vi "Progetto_AnalisiDimensionale_new.vi"() -> ()   [LabVIEW 2020]
panel:
  out "Write Error":errorcluster
  out "data":string[][](array[string])
  out "Read Error":errorcluster
  in  "Saving File Path":path
  out "Alarm":bool
  out "Length [mm]":dbl
  out "Speed [m/s]":dbl
  in  "Sensors_Distance [mm]":u32=101
  in  "Max_Time [ms]":u32
  in  "Trigger_S2":bool
  in  "Trigger_S1":bool
  in  "STOP":bool
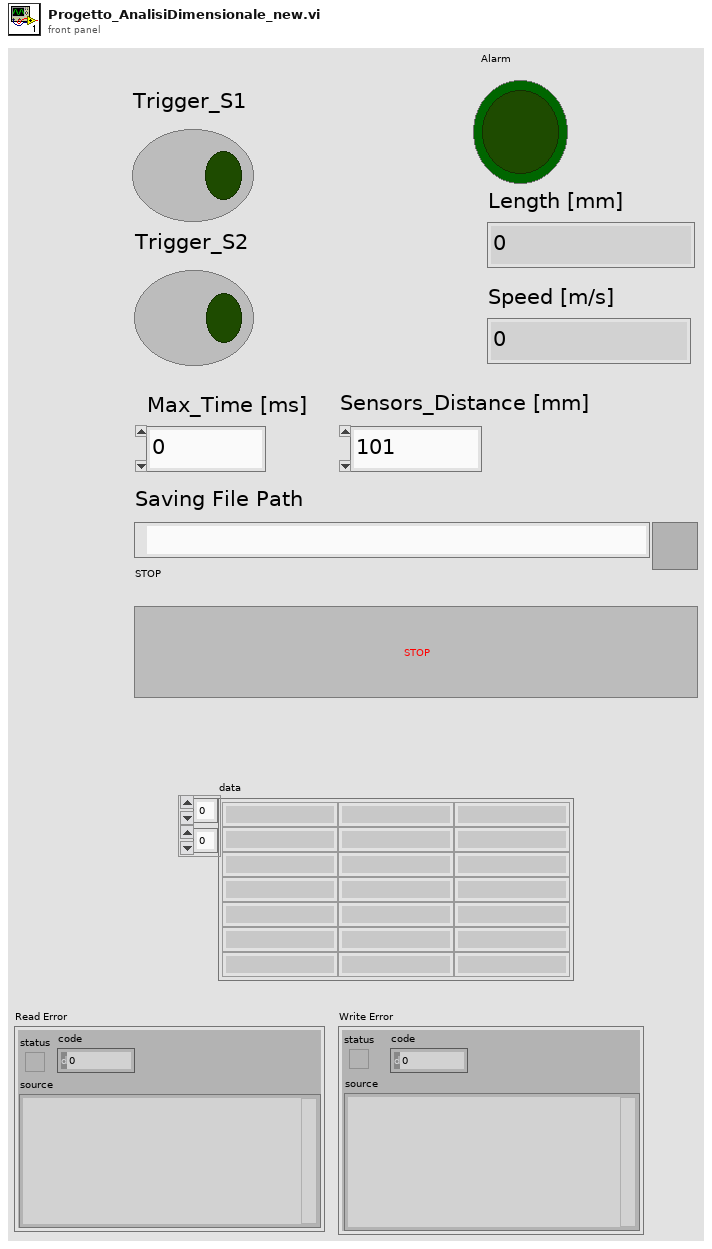
[diagram p1: front panel]
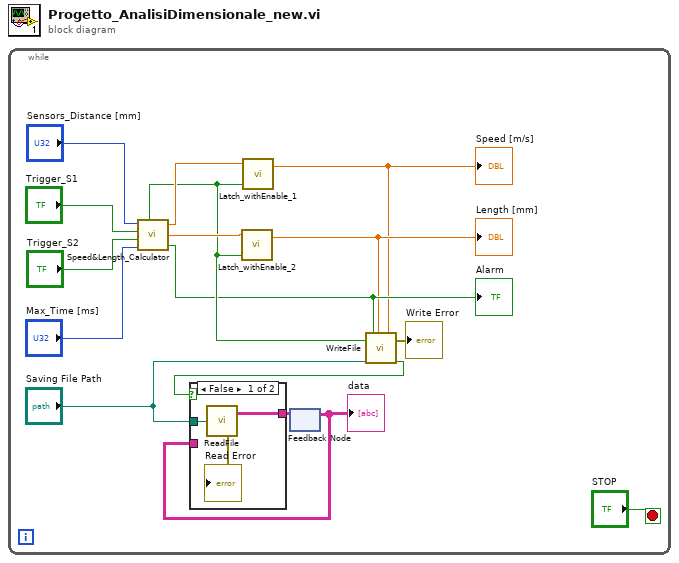
[diagram p0: block diagram]
diagram:
  n1 = while {
    stop <- "STOP" stop-if-true
    n2 = call "Speed&Length_Calculator.vi"("Sensors_Distance [mm]"="Sensors_Distance [mm]", "TriggerS1"="Trigger_S1", "TriggerS2"="Trigger_S2", "Max_Time [ms]"="Max_Time [ms]") -> ("Flag_EndMeasure"=w9:bool, "Speed [m/s]"=w11:dbl, "Length [mm]"=w10:dbl, "Alarm"=w8:bool)
    "Alarm" <- w8
    n3 = call "Latch_withEnable_2.vi"("Enable"=w9, "D"=w10) -> ("Q"=w7:dbl)  [unwired: 3 in]
    "Length [mm]" <- w7
    n4 = call "Latch_withEnable_1.vi"("Enable"=w9, "D"=w11) -> ("Q"=w6:dbl)  [unwired: 3 in]
    "Speed [m/s]" <- w6
    n5 = feedback #1() -> (w3:string[][])  [unwired: 1 in]
    "data" <- w3
    n6 = call "WriteFile.vi"("Enable"=w9, "Saving File Path"="Saving File Path", "Alarm"=w8, "Length [mm]"=w7, "Speed [m/s]"=w6) -> ("error out"=→"Write Error":errorcluster, "Saving Data"=w1:bool)  [unwired: 13 in]
    n7 = case shown="False" w1 {
      tunnel: "Saving File Path" -> [w19 _]
      tunnel: [w17 w20] -> w4
      tunnel: w3 -> [_ w20]
      frame False {
        n8 = call "ReadFile.vi"("template (empty)"=w19) -> ("data"=w17:string[][], "error out"=→"Read Error":errorcluster)
      }
      frame True {
      }
    }
    n9 = feedback-in #1(w4) -> ()
  }
